vi "Monitors_EPR_v00.vi"(8 "wfm":waveform(dbl)[](array[waveform]), 9 "Shot noise start":bool, 10 "Monitor Switches":T1, 11 "IIR filter specifications":T2={"Topology"=enum."Butterworth", "Type"=enum."Lowpass", "Order"=1, "Lower Fc"=100.0, "Upper Fc"=200.0, "PB Ripple"=1.0, "SB Attenuation"=60.0} {"PB Ripple" format="%0.2f"; "SB Attenuation" format="%0.2f"; "Lower Fc" format="%0.2p"; "Upper Fc" format="%0.2p"}) -> (0 "covariance":dbl, 1 "conditional variance A|B":dbl, 3 "Key Rate A|B":dbl)   [LabVIEW 2013]
uses:
  Strict Type Defs/Monitor switches.ctl
  <vilib>/Analysis/5stat.llb/RMS (DBL).vi
  <vilib>/Analysis/baseanly.llb/Mean (DBL).vi
  <vilib>/measure/macond.llb/IIR Filter for N Chan.vi
  shotnoise.vi
  <vilib>/measure/NI_MAPro.lvlib
  <vilib>/Analysis/NI_AALPro.lvlib
  <vilib>/Analysis/NI_AALBase.lvlib
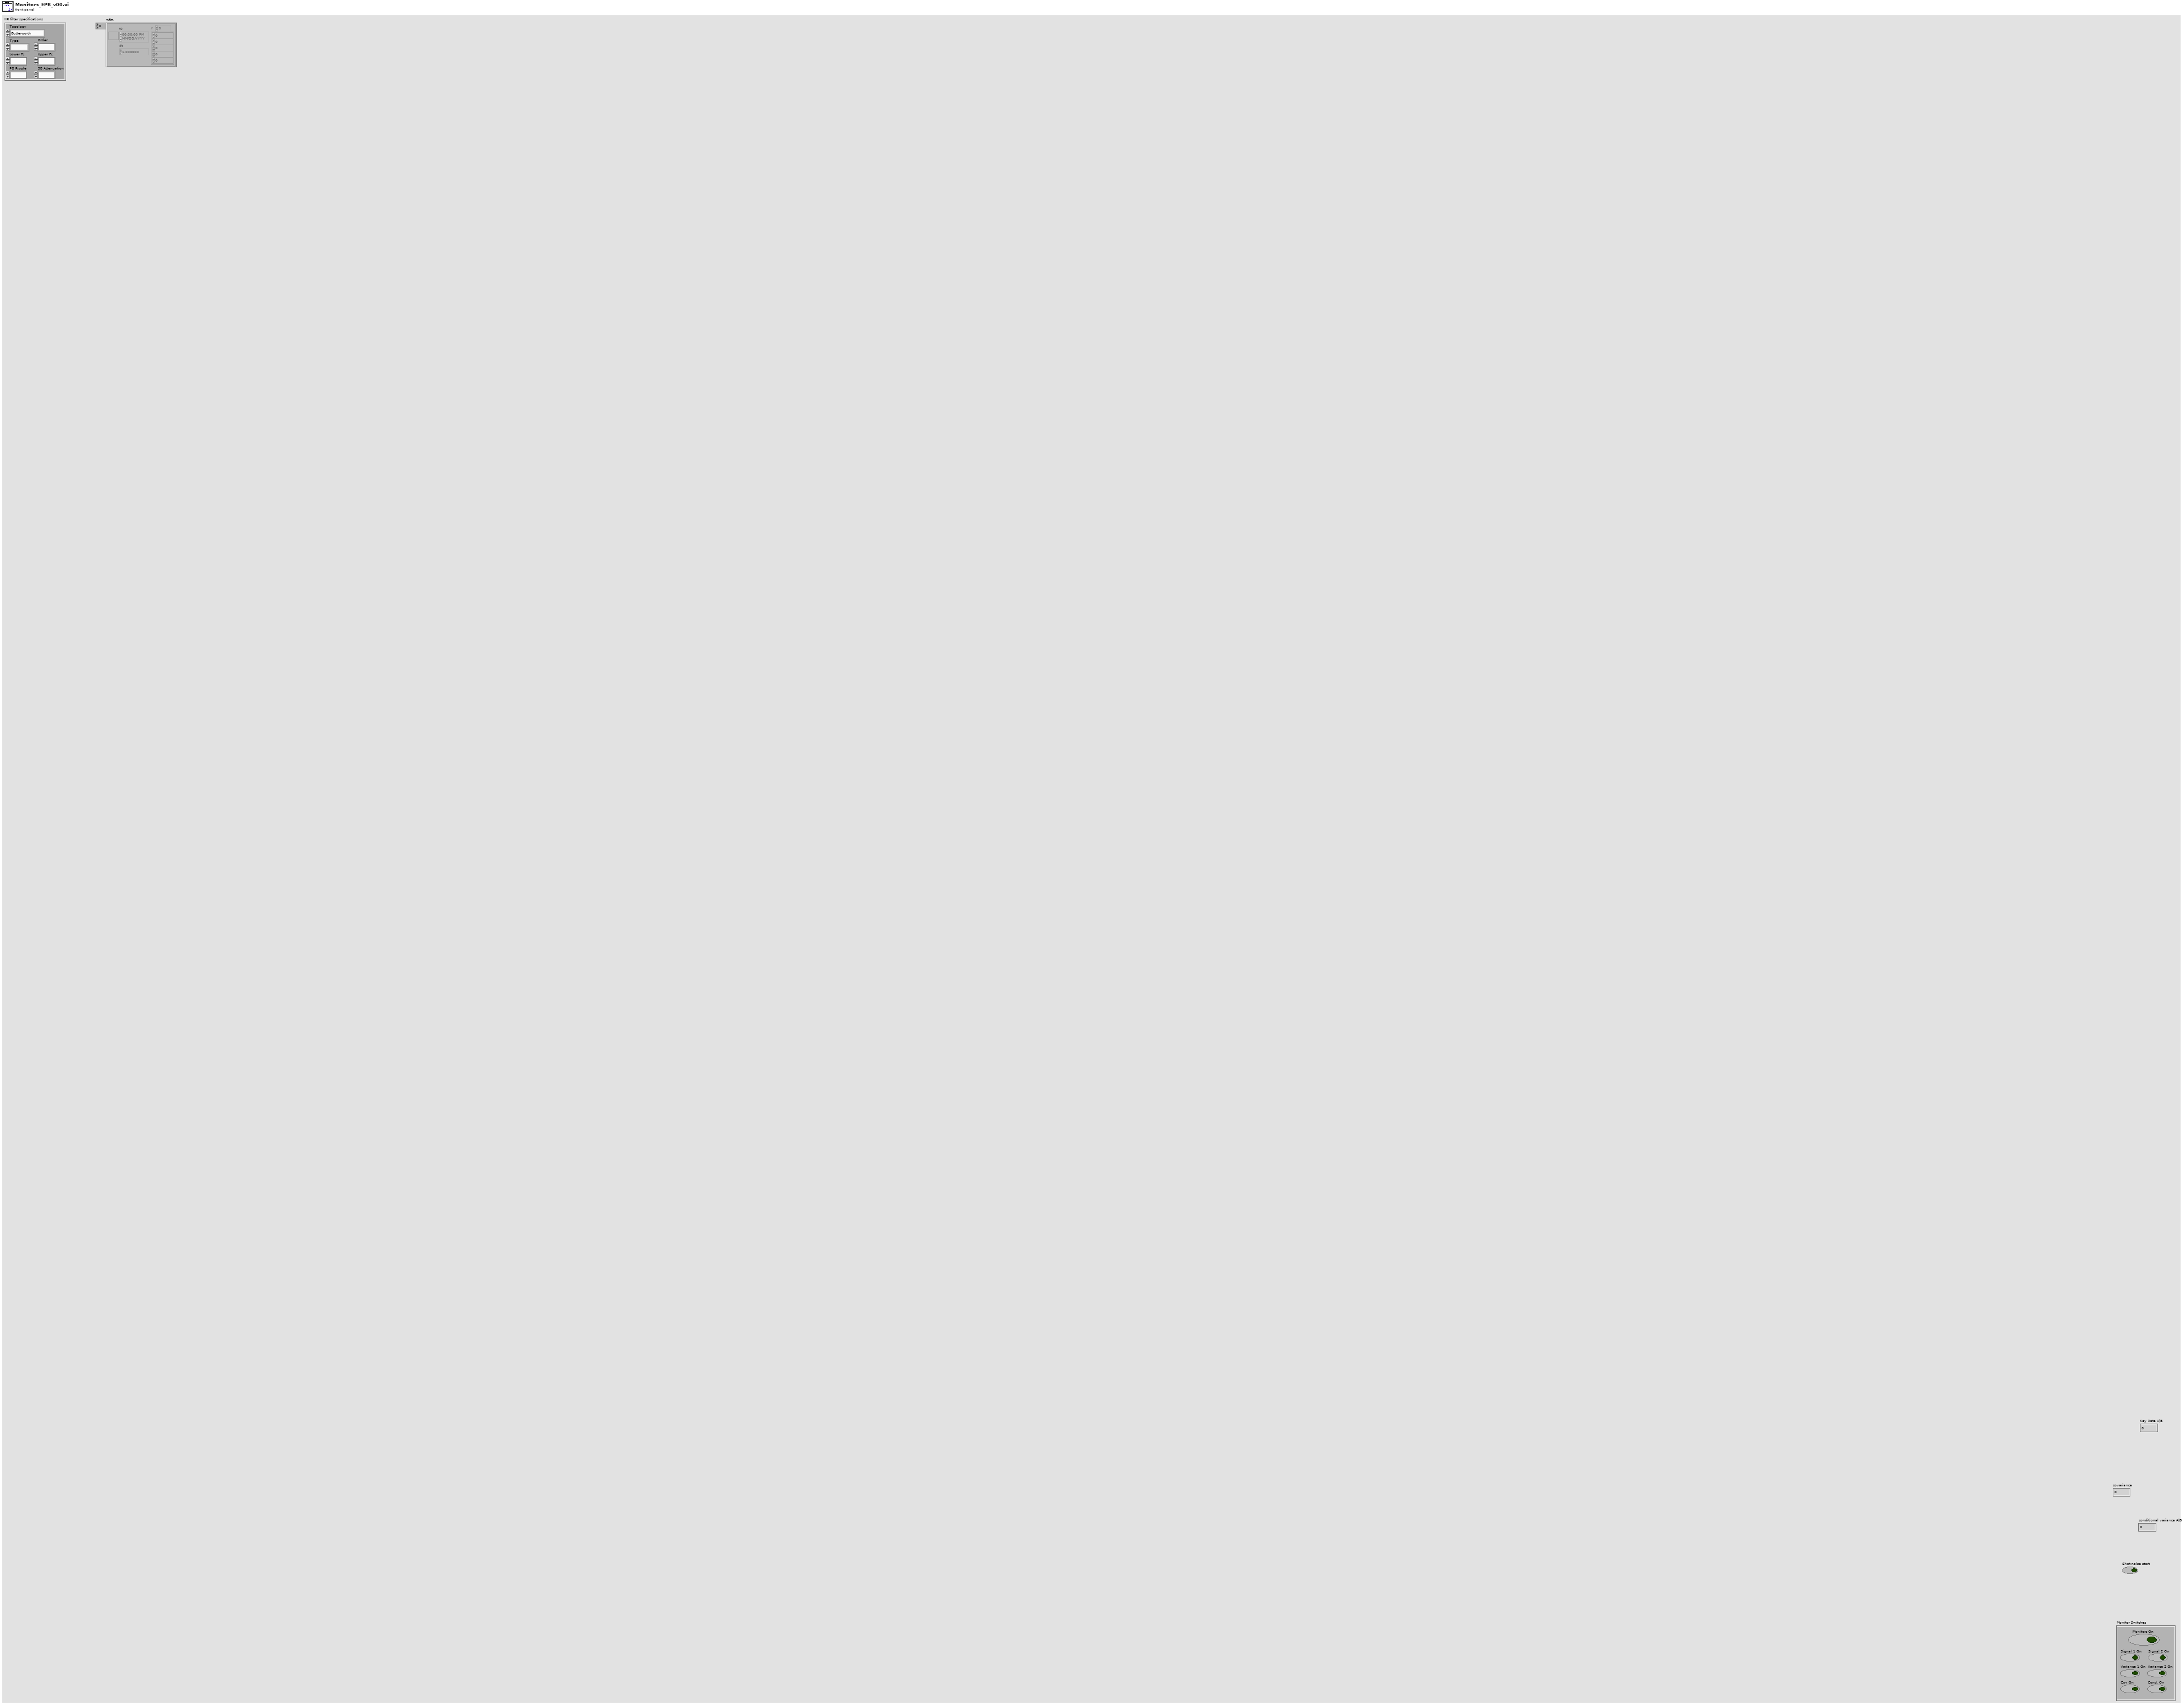
[diagram p1: front panel]
types:
  T1 = typedef "Monitor switches.ctl" = cluster{"Signal 1 On":bool, "Signal 2 On":bool, "Variance 1 On":bool, "Variance 2 On":bool, "Cov On":bool, "Cond. On":bool, "Monitors On":bool}
  T2 = cluster{"Topology":enum16{"Off", "Butterworth", "Chebyshev", "Inverse Chebyshev", "Elliptic", "Bessel"}, "Type":enum16{"Lowpass", "Highpass", "Bandpass", "Bandstop"}, "Order":i32, "Lower Fc":dbl, "Upper Fc":dbl, "PB Ripple":dbl, "SB Attenuation":dbl}
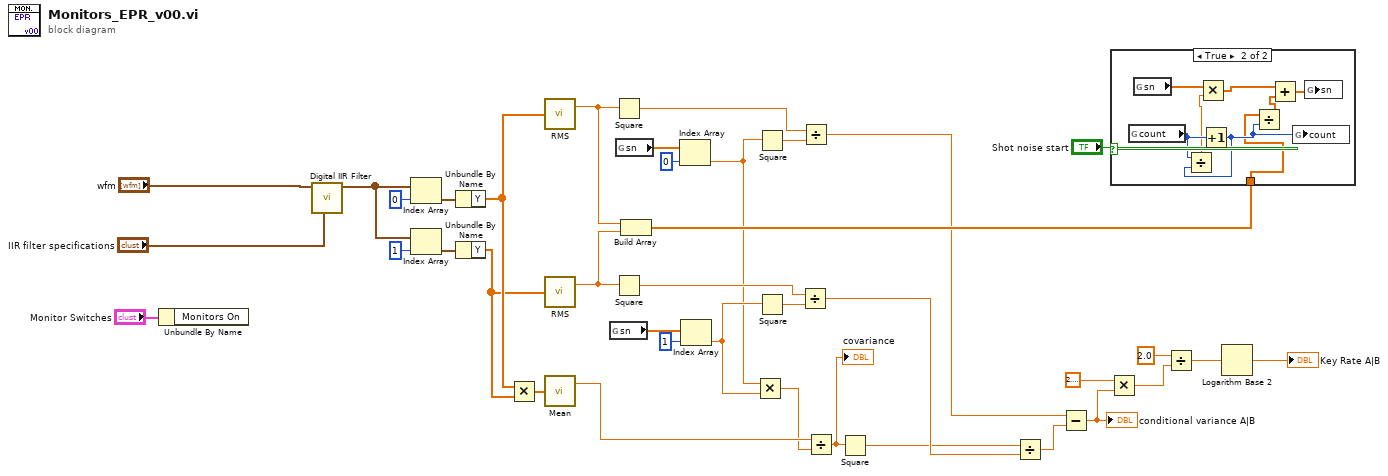
[diagram p0: block diagram]
diagram:
  n1 = Unbundle By Name("Monitor Switches") -> ()  [unwired: 1 out]
  n2 = call-poly <vilib>:"Digital IIR Filter.vi"("IIR filter specifications"="IIR filter specifications", "signal(s) in"="wfm") -> ("signal(s) out"=w7:waveform(dbl)[])  [unwired: 4 in, 5 out]
  n3 = Index Array(array=w7, index=0) -> (element=w10:waveform(dbl))
  n4 = Index Array(array=w7, index=1) -> (element=w15:waveform(dbl))
  n5 = Unbundle By Name(w10) -> ("Y"=w34:dbl[])
  n6 = Unbundle By Name(w15) -> ("Y"=w29:dbl[])
  n7 = Multiply(x=w34, y=w29) -> (x*y=w32:dbl[])
  n8 = call-poly <vilib>:"RMS.vi"("X"=w34) -> ("rms value"=w27:dbl)  [unwired: 1 out]
  n9 = call-poly <vilib>:"RMS.vi"("X"=w29) -> ("rms value"=w30:dbl)  [unwired: 1 out]
  n10 = call-poly <vilib>:"Mean.vi"("X"=w32) -> ("mean"=w33:dbl)  [unwired: 1 out]
  n11 = global read "shotnoise.vi" "sn"() -> (w13:dbl[])
  n12 = Square(x=w27) -> (x^2=w28:dbl)
  n13 = Square(x=w30) -> (x^2=w31:dbl)
  n14 = global read "shotnoise.vi" "sn"() -> (w12:dbl[])
  n15 = Build Array(w27, w30) -> (w26:dbl[])
  n16 = Index Array(array=w12, index=0) -> (element=w22:dbl)
  n17 = Index Array(array=w13, index=1) -> (element=w23:dbl)
  n18 = Multiply(x=w22, y=w23) -> (x*y=w24:dbl)
  n19 = Square(x=w22) -> (x^2=w19:dbl)
  n20 = Square(x=w23) -> (x^2=w21:dbl)
  n21 = Divide(x=w31, y=w21) -> (x/y=w25:dbl)
  n22 = Divide(x=w28, y=w19) -> (x/y=w20:dbl)
  n23 = Divide(x=w33, y=w24) -> (x/y=w35:dbl)
  "covariance" <- w35
  n24 = Square(x=w35) -> (x^2=w17:dbl)
  n25 = Divide(x=w17, y=w25) -> (x/y=w18:dbl)
  n26 = Subtract(x=w20, y=w18) -> (x-y=w6:dbl)
  "conditional variance A|B" <- w6
  n27 = Multiply(x=2.718281828459045, y=w6) -> (x*y=w3:dbl)
  n28 = case shown="True" "Shot noise start" {
    tunnel: w26 -> [_ w40]
    frame False {
    }
    frame True {
      n29 = global read "shotnoise.vi" "count"() -> (w45:i64)
      n30 = global read "shotnoise.vi" "sn"() -> (w44:dbl[])
      n31 = Increment(x=w45) -> (x+1=w41:i64)
      n32 = Divide(x=w45, y=w41) -> (x/y=w43:dbl)
      n33 = Multiply(x=w44, y=w43) -> (x*y=w42:dbl[])
      n34 = Divide(x=w40, y=w41) -> (x/y=w39:dbl[])
      n35 = Add(x=w42, y=w39) -> (x+y=w46:dbl[])
      n36 = global write "shotnoise.vi" "count"(w41) -> ()
      n37 = global write "shotnoise.vi" "sn"(w46) -> ()
    }
  }
  n38 = Divide(x=2.0, y=w3) -> (x/y=w2:dbl)
  n39 = Logarithm Base 2(1:w2) -> (0:→"Key Rate A|B":dbl)
